vi "开始界面.vi"() -> ()   [LabVIEW 2018]
panel:
  in  "VI路径":path=path "C:/Users/acer/Desktop/地学虚拟仪器/动态界面.vi"
  in  "登录":bool
  in  "用户名":string
  in  "密码":string
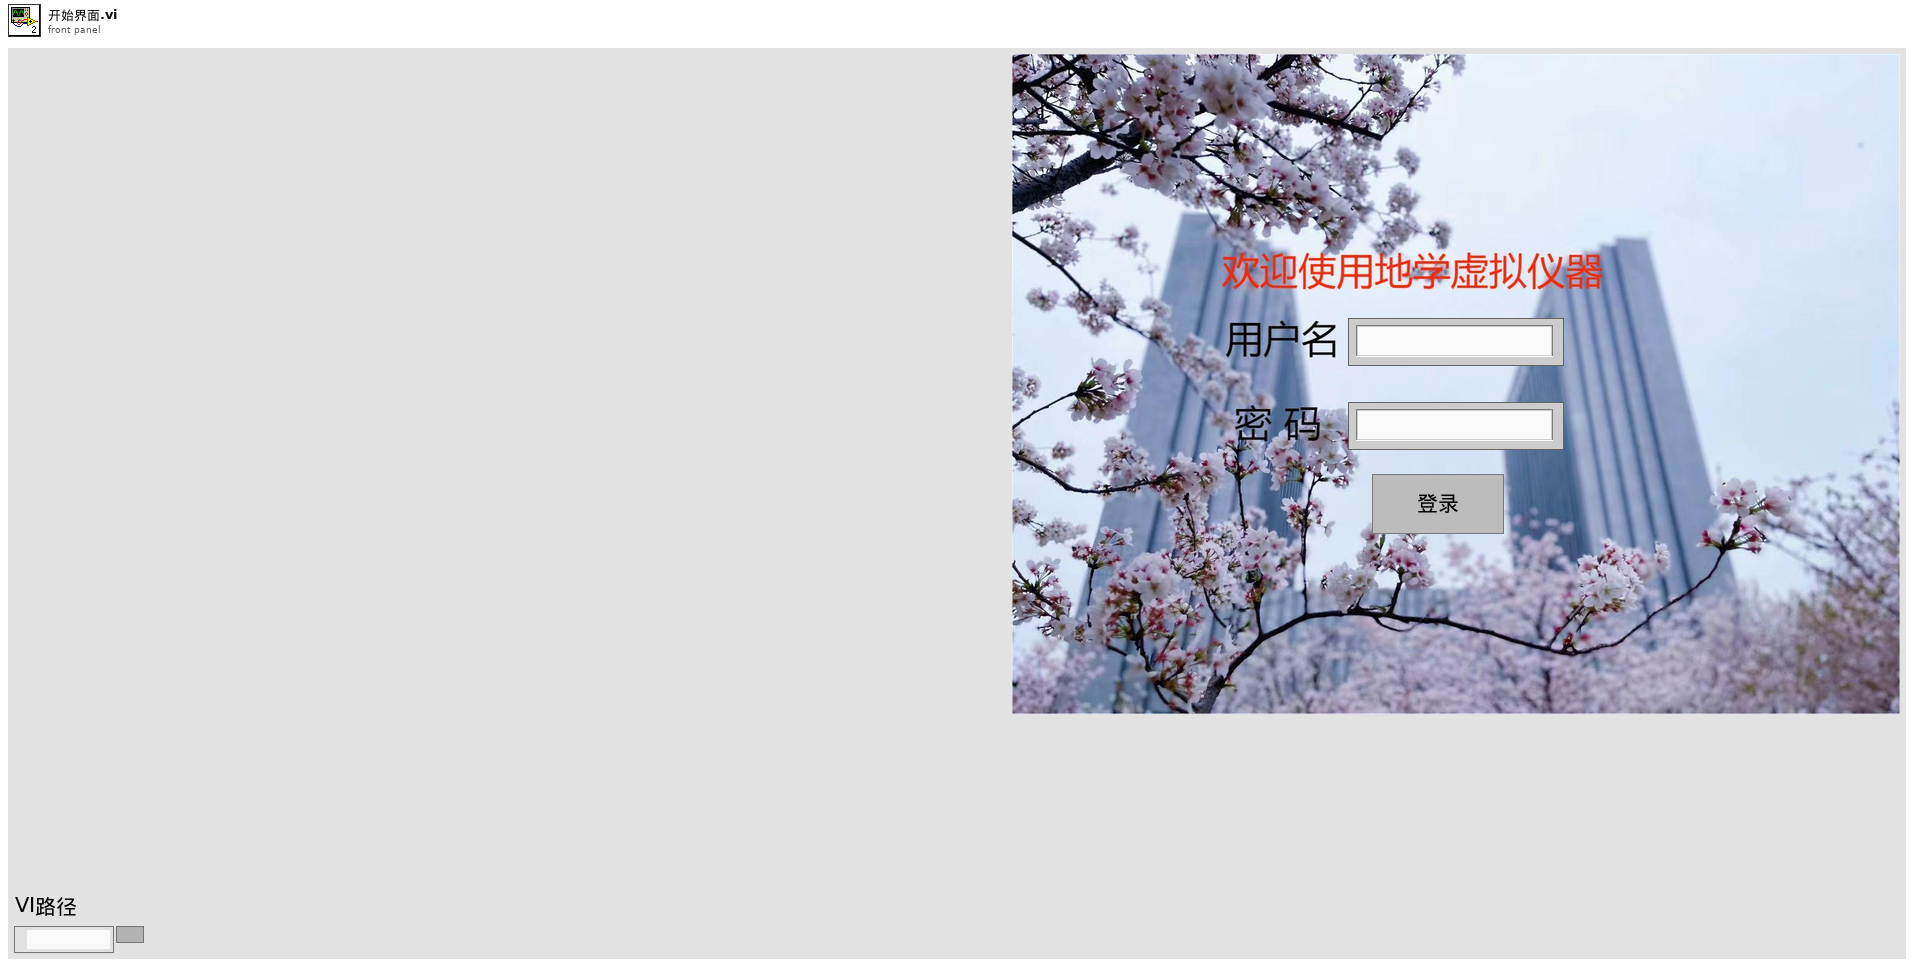
[diagram p1: front panel]
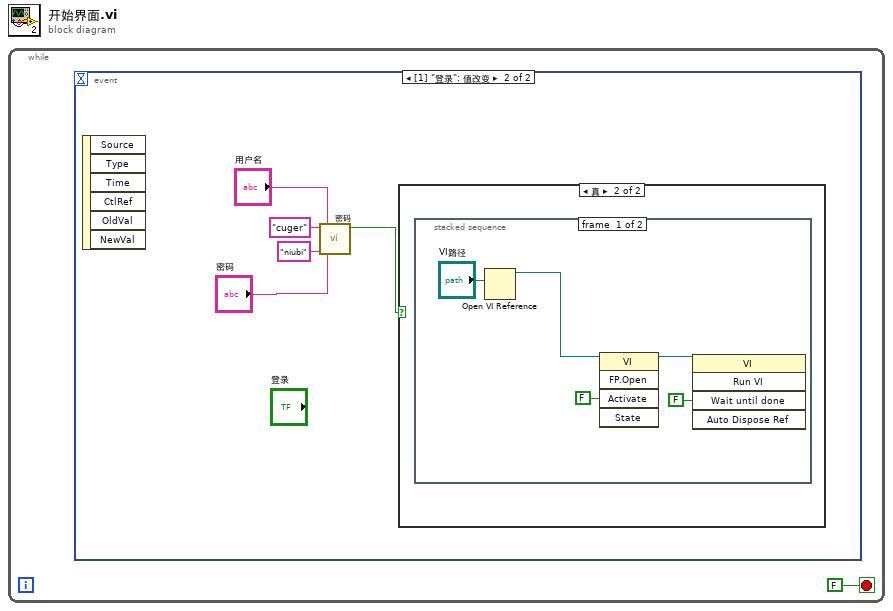
[diagram p0: block diagram]
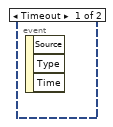
[diagram p2: hidden frame]
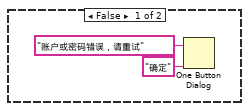
[diagram p3: hidden frame]
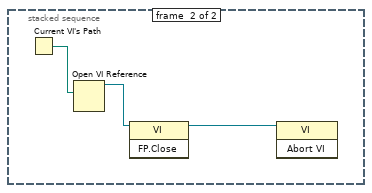
[diagram p4: hidden frame]
diagram:
  n1 = while {
    stop <- FALSE stop-if-true
    n2 = event shown="[1] \"登录\": 值改变" {
      selector: _ -> [_ _]
      dyn-events: _ -> [_ _]
      timeout: _ -> [_ _]
      event Timeout {
        n3 = event-data() -> ()  [unwired: 1 in, 3 out]
      }
      event "登录": Value Change {
        n4 = event-data() -> ()  [unwired: 1 in, 6 out]
        n5 = call "密码.vi"("字符串 2"="niubi", "密码"="密码", "用户名"="用户名", "字符串"="cuger") -> ("x与y？"=w4:bool)  [unwired: 3 in]
        n6 = case shown="真" w4 {
          frame False {
            n7 = One Button Dialog(message="账户或密码错误，请重试" ("消息"), button name ("OK")="确定" ("按钮名称（“确定”）")) -> ()  [unwired: 1 out]
          }
          frame True {
            n8 = stacked-sequence {
              frame #0 {
                n9 = Open VI Reference(vi path="VI路径") -> (vi reference=w12:refnum<vi>)  [unwired: 5 in, 1 out]
                n10 = invoke class="VI" method="FP.Open"(reference=w12, "Activate"=FALSE ("激活？")) -> (reference out=w13:refnum<vi>)  [unwired: 3 in, 4 out]
                n11 = invoke class="VI" method="Run VI"(reference=w13, "Wait until done"=FALSE ("结束前等待")) -> ()  [unwired: 3 in, 5 out]
              }
              frame #1 {
                n12 = Current VI's Path() -> (path=w16:path)
                n13 = Open VI Reference(vi path=w16) -> (vi reference=w15:refnum<vi>)  [unwired: 5 in, 1 out]
                n14 = invoke class="VI" method="FP.Close"(reference=w15) -> (reference out=w14:refnum<vi>)  [unwired: 2 in, 2 out]
                n15 = invoke class="VI" method="Abort VI"(reference=w14) -> ()  [unwired: 2 in, 3 out]
              }
            }
          }
        }
      }
    }
  }
